vi "getPolarity.vi"(0 "Controller in":refnum<class "_Controller.lvclass">, 2 "axis (def=X)":T3, 5 "error in (no error)":errorcluster) -> (14 "Controller out":refnum<class "_Controller.lvclass">, 16 "polarity_items (out)":T1[](array[typedef]), 19 "error out":errorcluster)   [LabVIEW 2013, in "classes.lvlib" / "_Controller.lvclass"]
doc: "Get the current Polarity Values for a given axis. For single axis applications, axis need not be specified.\n\nProduced By:\n\n<B>Kod Integrations, LLC</B>\n4835 Marianne Drive\nMount Airy, MD 21771\nhttp://www.kodintegrations.com\nemail: info@kodintegrations.com\nphone: (240) 687-1288"
uses:
  _Controller.lvclass
  common/controls/axis.ctl
  common/controls/polarity_item.ctl
  common/controls/polarity.ctl
  libraries/common.lvlib
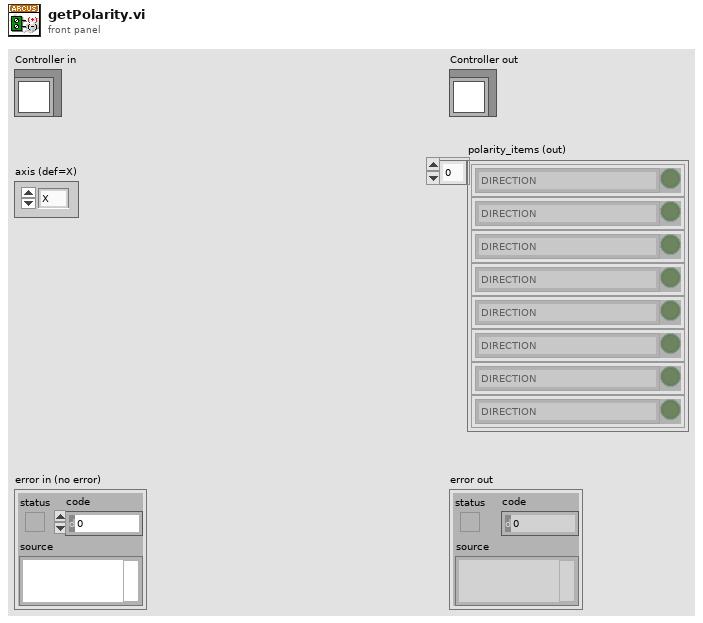
[diagram p1: front panel]
types:
  T1 = typedef "common.lvlib/polarity_item.ctl" = cluster{"item":T2, "status":bool}
  T2 = typedef "common.lvlib/polarity.ctl" = enum16{"DIRECTION", "LIMIT", "HOME", "DIG_OUT", "DIG_IN", "ENABLE_OUT", "JUMP_ERR", "LATCH", "Z-CHAN_INDEX", "ENCODER_DECODING:1X", "ENCODER_DECODING:2X", "ENCODER_DECODING:4X", "ALARM", "STANDALONE_ERR", "-", "<reserved/nc>"}
  T3 = typedef "common.lvlib/axis.ctl" = enum16{"X", "Y", "Z", "U"}
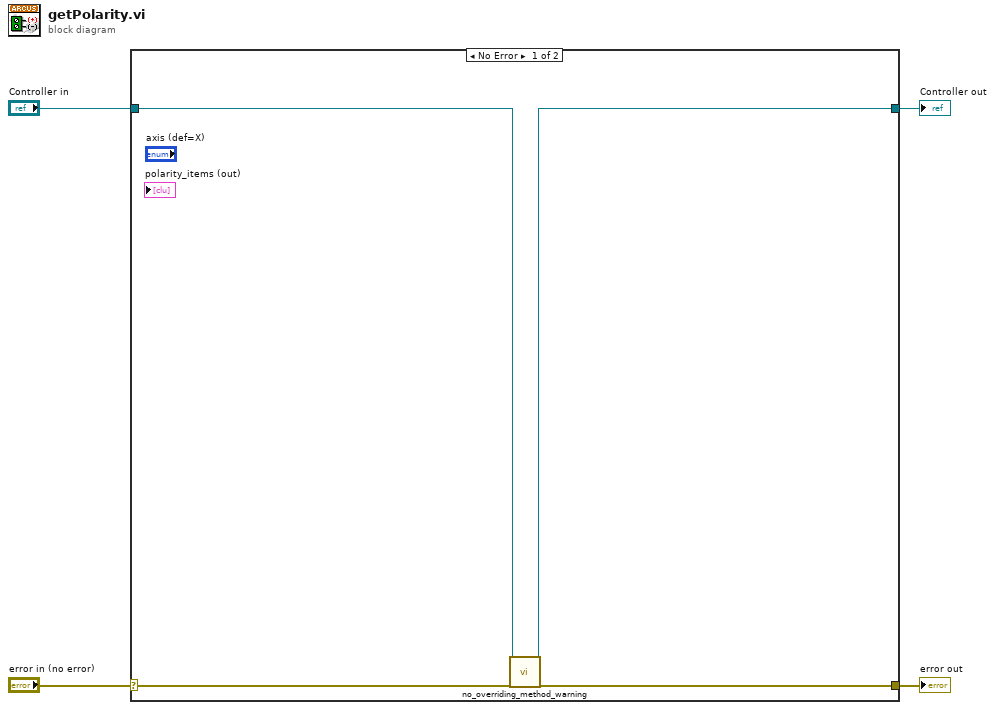
[diagram p0: block diagram]
diagram:
  n1 = case shown="No Error" "error in (no error)" {
    selector: "error in (no error)" -> [w8 w10]
    tunnel: [w7 w10] -> w3
    tunnel: [w5 w9] -> w1
    tunnel: "Controller in" -> [w6 w9]
    frame No Error {
      n2 = call "no_overriding_method_warning.vi"("Controller (in)"=w6, "error in (no error)"=w8) -> ("Controller (out)"=w5:refnum<class "_Controller.lvclass">, "error out"=w7:errorcluster)  [unwired: 15 in, 1 out]
    }
    frame Error {
    }
  }
  "error out" <- w3
  "Controller out" <- w1
